vi "WaitInId.vi"(1 "IO_Input":i32, 2 "Wait?":bool=TRUE, 3 "Status":bool, 5 "error in":errorcluster, 8 "CardNum":i32) -> (14 "StatusOut":bool, 17 "TimeOut":bool, 19 "error Out":errorcluster)   [LabVIEW 2019]
uses:
  global/IO_FlagGB.vi
  IO_Class/IOCard.lvclass
panel:
  in  "time(0.1)":i32=100
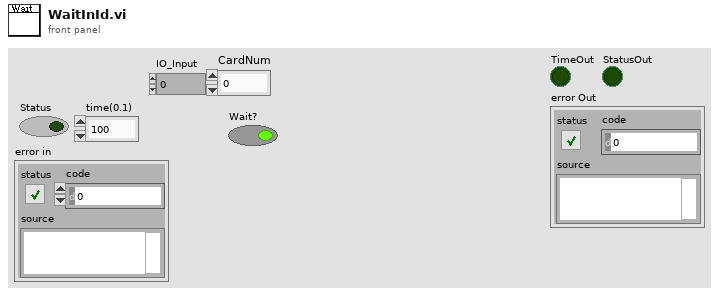
[diagram p1: front panel]
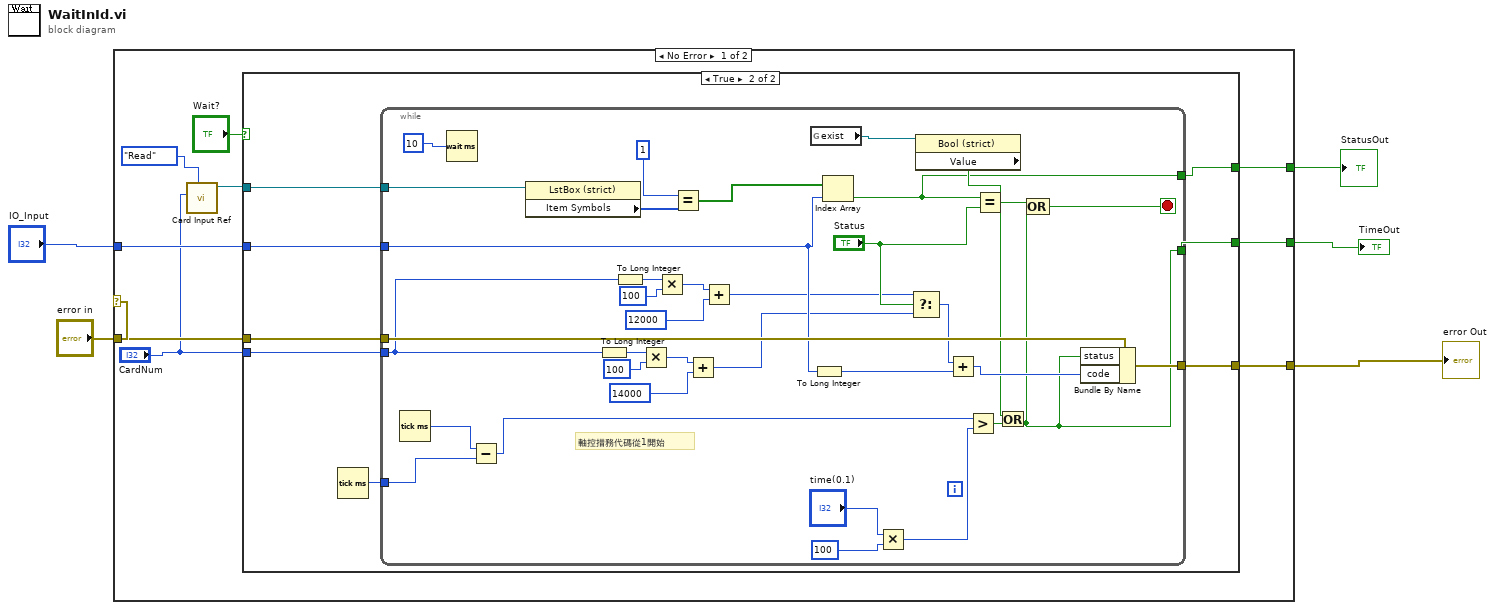
[diagram p0: block diagram]
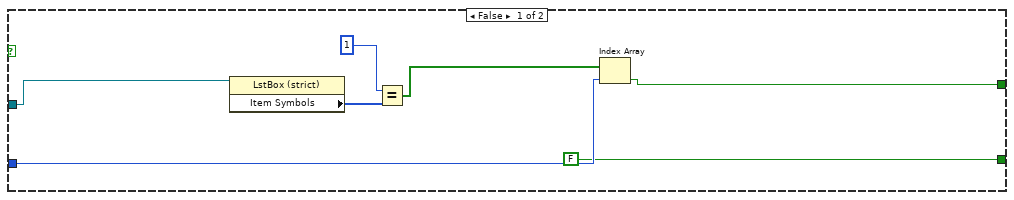
[diagram p2: hidden frame]
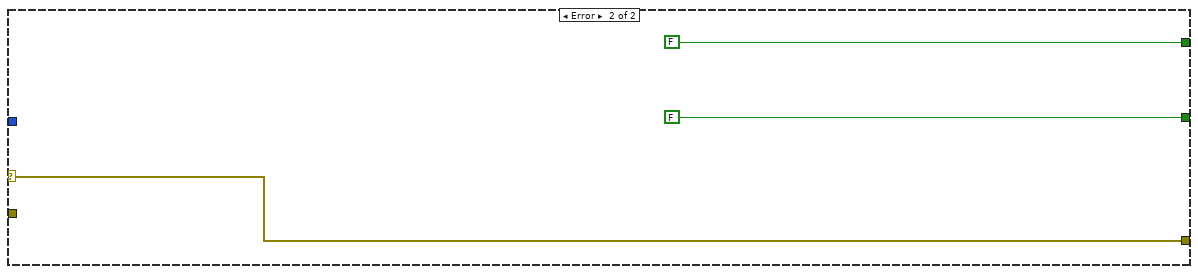
[diagram p3: hidden frame]
diagram:
  n1 = case shown="No Error" "error in" {
    selector: "error in" -> [_ w67]
    tunnel: [w14 FALSE] -> w5
    tunnel: "error in" -> [w13 _]
    tunnel: [w12 w67] -> w4
    tunnel: [w11 FALSE ("Boolean")] -> w2
    tunnel: "IO_Input" -> [w9 _]
    frame No Error {
      n2 = call "Card Input Ref.vi"("Action"=enum16{"Initial", "Write", "Read", "Release"}."Read", "CardIndex"="CardNum") -> ("RefOut"=w7:refnum<vi>)  [unwired: 8 in, 1 out]
      n3 = case shown="True" "Wait?" {
        tunnel: [FALSE w29] -> w14
        tunnel: w13 -> [_ w28]
        tunnel: [_ w27] -> w12
        tunnel: [w20 w26] -> w11
        tunnel: w9 -> [w21 w25]
        tunnel: w7 -> [w16 w23]
        tunnel: "CardNum" -> [_ w22]
        frame False {
          n4 = property class="LstBox (strict)"(reference=w16) -> ("Item Symbols"=w18:i32[])  [unwired: 1 in, 2 out]
          n5 = Equal?(x=1, y=w18) -> (x = y?=w15:bool[])
          n6 = Index Array(array=w15, index=w21) -> (element=w20:bool)
        }
        frame True {
          n7 = Tick Count (ms)() -> (millisecond timer value=w24:u32)
          n8 = while {
            tunnel: [w55] -> w29
            tunnel: w28 -> [w62]
            tunnel: [w59] -> w27
            tunnel: [w31] -> w26
            tunnel: w25 -> [w53]
            tunnel: w24 -> [w37]
            tunnel: w23 -> [w35]
            tunnel: w22 -> [w30]
            stop <- w64 stop-if-true
            # "軸控措務代碼從1開始"
            n9 = Tick Count (ms)() -> (millisecond timer value=w38:u32)
            n10 = Wait (ms)(milliseconds to wait=u32 10) -> ()  [unwired: 1 out]
            n11 = Subtract(x=w38, y=w37) -> (x-y=w36:u32)
            n12 = property class="LstBox (strict)"(reference=w35) -> ("Item Symbols"=w34:i32[])  [unwired: 1 in, 2 out]
            n13 = To Long Integer(number=w30) -> (32bit integer=w43:i32)
            n14 = To Long Integer(number=w30) -> (32bit integer=w51:i32)
            n15 = Multiply(x=w43, y=100) -> (x*y=w45:i32)
            n16 = Multiply(x=w51, y=100) -> (x*y=w49:i32)
            n17 = Equal?(x=1, y=w34) -> (x = y?=w32:bool[])
            n18 = Add(x=w45, y=14000) -> (x+y=w42:i32)
            n19 = Add(x=w49, y=12000) -> (x+y=w47:i32)
            n20 = global read "IO_FlagGB.vi" "exist"() -> (w52:refnum<vi>)
            n21 = To Long Integer(number=w53) -> (32bit integer=w56:i32)
            n22 = Index Array(array=w32, index=w53) -> (element=w31:bool)
            n23 = Multiply(x="time(0.1)", y=u32 100 ("milliseconds to wait")) -> (x*y=w39:u32)
            n24 = Select(t=w47, s="Status", f=w42) -> (s? t:f=w57:i32)
            n25 = property class="Bool (strict)"(reference=w52) -> ("Value"=w54:bool)  [unwired: 1 in, 2 out]
            n26 = Add(x=w57, y=w56) -> (x+y=w60:i32)
            n27 = Greater?(x=w36, y=w39) -> (0:w61:bool)
            n28 = Equal?(x=w31, y="Status") -> (x = y?=w63:bool)
            n29 = Or(x=w54, y=w61) -> (x .or. y?=w55:bool)
            n30 = Compound Arithmetic op=OR(w63, w55) -> (w64:bool)
            n31 = Bundle By Name(cluster=w62, "status"=w55, "code"=w60) -> (w59:errorcluster)
          }
        }
      }
    }
    frame Error {
    }
  }
  "TimeOut" <- w5
  "error Out" <- w4
  "StatusOut" <- w2
